vi "Ejercicio 2.1.vi"() -> ()   [LabVIEW 2013]
panel:
  out "Waveform Graph":dbl[](graph)
  in  "Amplitud":dbl
  in  "Frecuencia":i32
  in  "Cantidad de muestras":i32=20
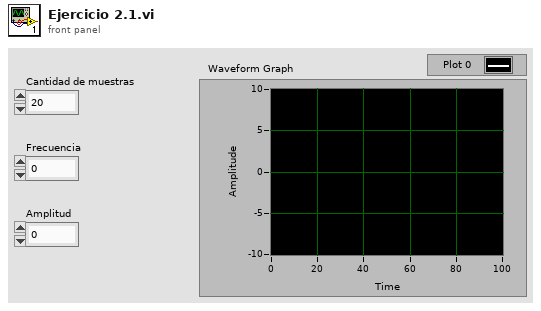
[diagram p1: front panel]
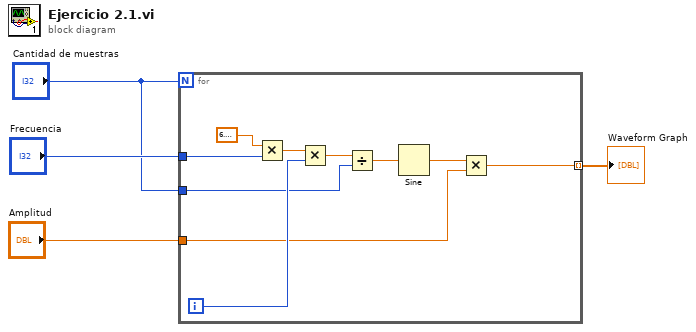
[diagram p0: block diagram]
diagram:
  n1 = for {
    N: "Cantidad de muestras" -> [_]
    tunnel: "Frecuencia" -> [w12]
    tunnel: "Amplitud" -> [w7]
    tunnel: [w6] -> w2 mode=indexing
    tunnel: "Cantidad de muestras" -> [w5]
    i -> [w11]
    n2 = Multiply(x=6.283185307179586, y=w12) -> (x*y=w14:dbl)
    n3 = Multiply(x=w14, y=w11) -> (x*y=w10:dbl)
    n4 = Divide(x=w10, y=w5) -> (x/y=w9:dbl)
    n5 = Sine(x=w9) -> (sin(x)=w8:dbl)
    n6 = Multiply(x=w8, y=w7) -> (x*y=w6:dbl)
  }
  "Waveform Graph" <- w2
